vi "CheckData.vi"() -> ()   [LabVIEW 2019]
uses:
  Communication/TypeDef/#TypeDef_PropertiesToSave.ctl
  App/Global_Freq.vi
  <vilib>/Analysis/NI_AALBase.lvlib
  <vilib>/Analysis/baseanly.llb/Mean (DBL).vi
  <vilib>/Analysis/NI_AALPro.lvlib
  <vilib>/Analysis/5stat.llb/RMS (DBL).vi
  <vilib>/gmath/NI_Gmath.lvlib
panel:
  in  "Calc":bool
  in  "Tab Control":enum32{"Page 1", "Page 2", "Page 3"}(tab)
  out "Mean":dbl[][](graph)
  out "Corelation R^2":dbl[][](graph)
  out "RMS":dbl[][](graph)
  out "Corelation R":dbl[][](graph)
  out "Step":dbl format="%#_13g"
  out "TEST":cluster{"f0":dbl, "df":dbl, "magnitude":dbl[]}[](graph) caption="Power Spectrum TEST"
  out "POMIAR":cluster{"f0":dbl, "df":dbl, "magnitude":dbl[]}[](graph) caption="Power Spectrum POMIAR"
  out "Z":dbl[][](graph)
  out "Y":dbl[][](graph)
  out "X":dbl[][](graph)
  in  "Test Offset":i32
  in  "Pomiar Offset":i32
  in  "file path":path
  out "Poperties":T1
  in  "stop":bool
  in  "Lista_Archive":i32(listbox) caption="Lista pomiarów"
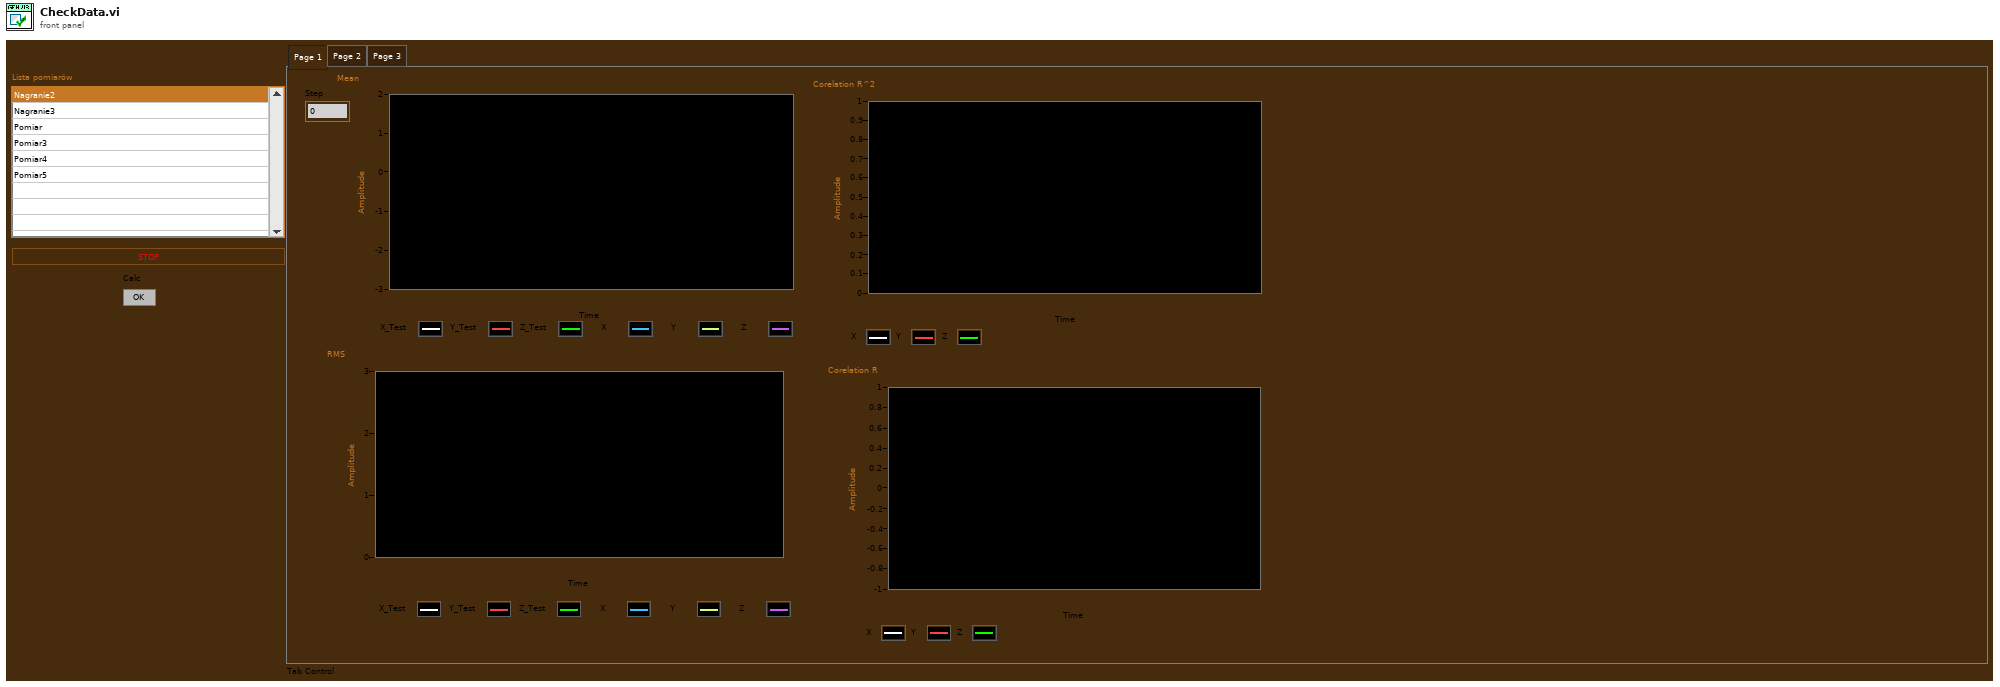
[diagram p1: front panel]
types:
  T1 = typedef "#TypeDef_PropertiesToSave.ctl" = cluster{"RMS values":dbl[], "Max":dbl[], "Min":dbl[], "A(8)":dbl[], "t":dbl, "A(8) Axis":dbl, "Aw":dbl[], "Ak 30min":dbl, "Ak_axis":i32, "Spec":cluster{"f0":dbl, "df":dbl, "magnitude":dbl[]}[]}
  T2 = enum16{"open", "open or create", "create or replace", "create", "open (read-only)"}
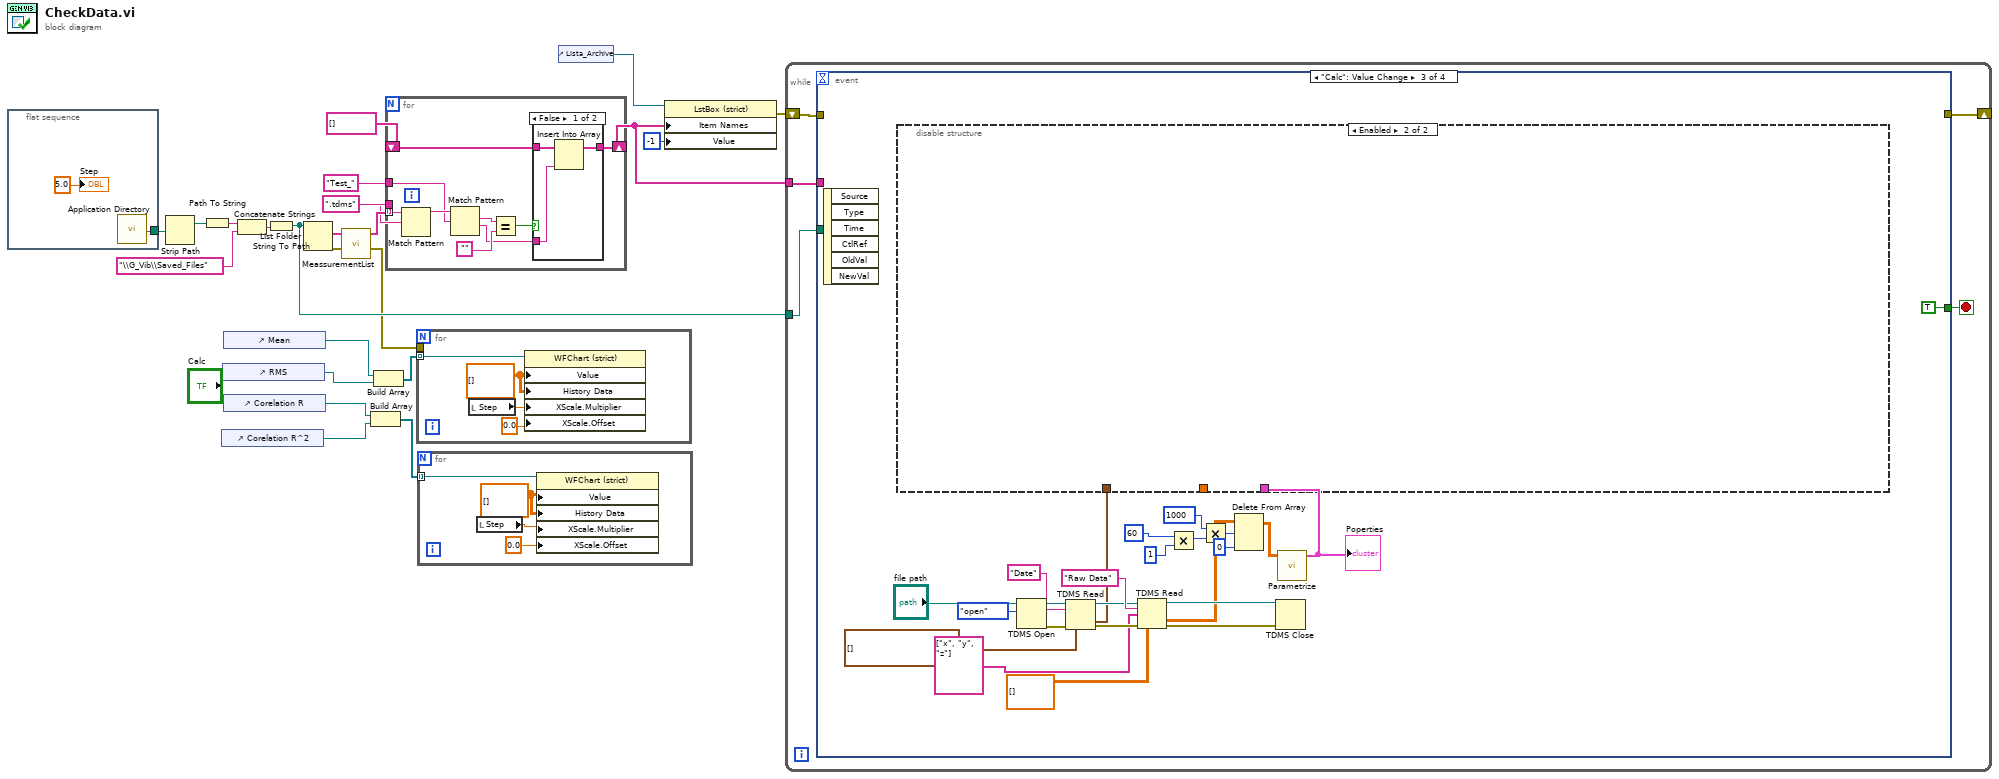
[diagram p0: block diagram]
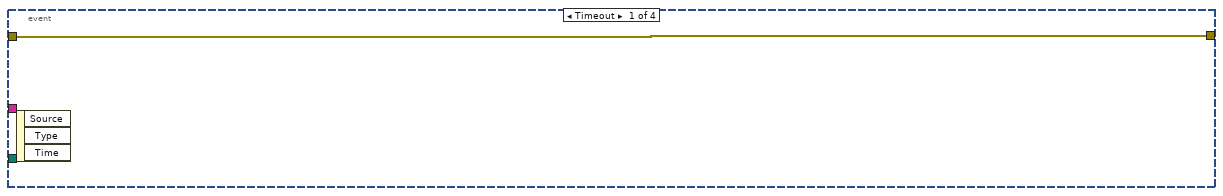
[diagram p2: hidden frame]
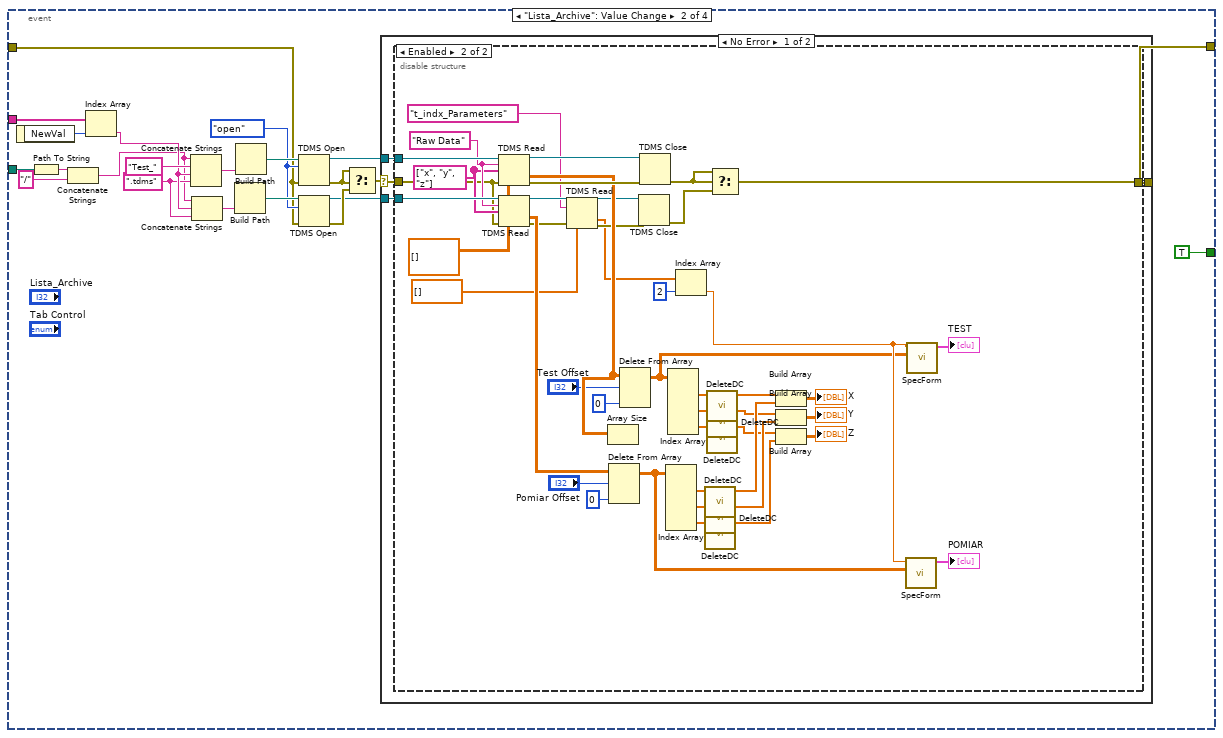
[diagram p3: hidden frame]
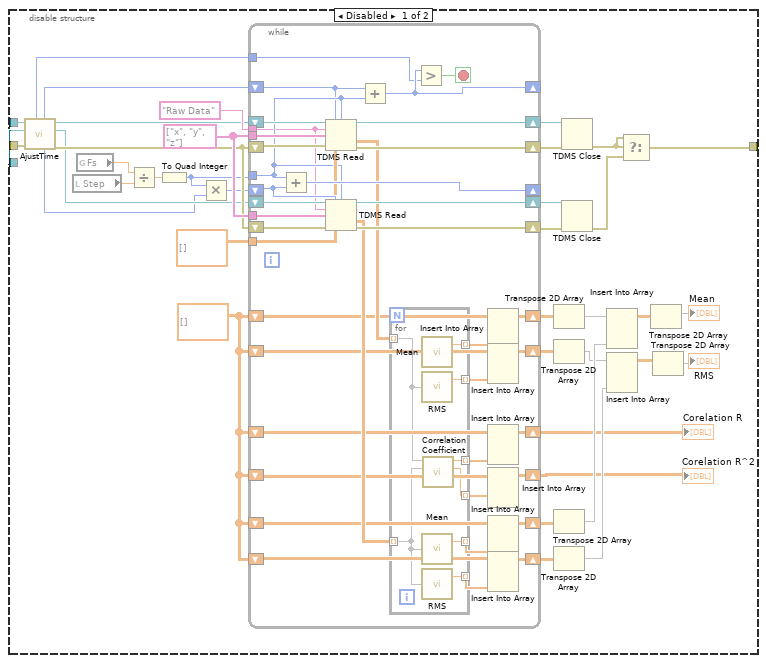
[diagram p4: hidden frame]
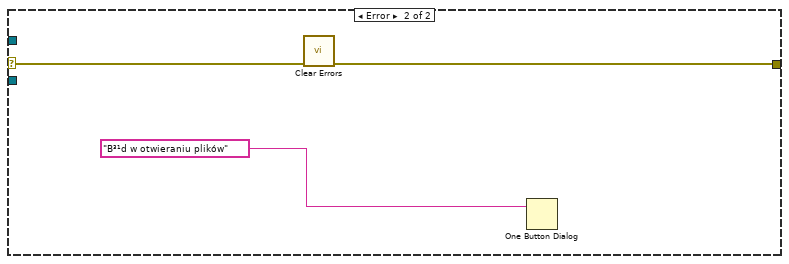
[diagram p5: hidden frame]
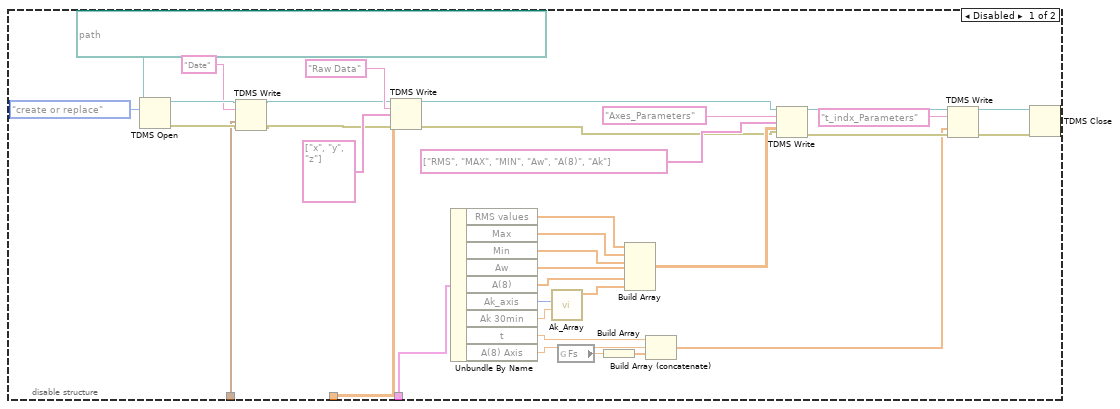
[diagram p6: hidden frame]
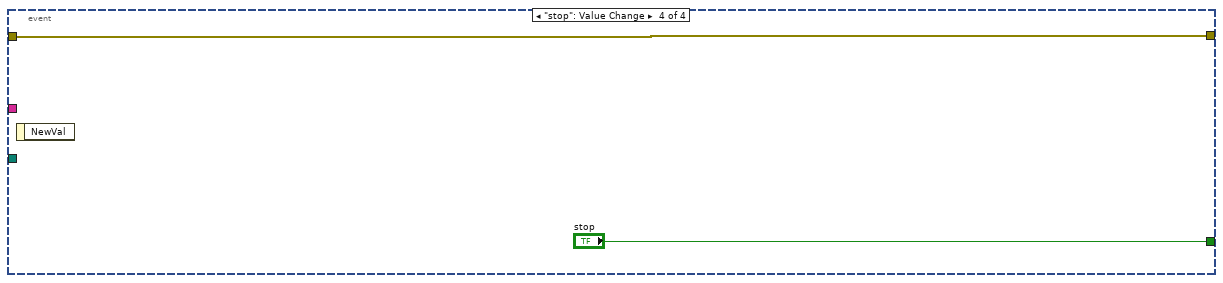
[diagram p7: hidden frame]
diagram:
  n1 = flat-sequence {
    tunnel: [w24] -> w2
    frame #0 {
      n2 = call <vilib>:"Application Directory.vi"() -> ("Application Directory"=w24:path)
      "Step" <- 5.0 ("Step")
    }
  }
  n3 = Strip Path(path=w2) -> (stripped path=w22:path)  [unwired: 1 out]
  n4 = Path To String(path=w22) -> (string=w21:string)
  n5 = control-ref of="Corelation R^2"() -> (w6:refnum<vi>)
  n6 = control-ref of="RMS"() -> (w8:refnum<vi>)
  n7 = control-ref of="Mean"() -> (w9:refnum<vi>)
  n8 = control-ref of="Corelation R"() -> (w7:refnum<vi>)
  n9 = Concatenate Strings(w21, "\\G_Vib\\Saved_Files" ("string")) -> (w20:string)
  n10 = String To Path(string=w20) -> (path=w10:path)
  n11 = List Folder(path=w10) -> (filenames=w18:string[], error out=w3:errorcluster)  [unwired: 3 in, 2 out]
  n12 = call "MeassurementList.vi"("filenames"=w18) -> ("ListaPomiarów"=w17:string[])  [unwired: 10 in]
  n13 = Build Array(w7, w6) -> (w4:refnum<vi>[])
  n14 = Build Array(w9, w8) -> (w5:refnum<vi>[])
  n15 = for {
    tunnel: w17 -> [w34] mode=indexing
    tunnel: ".tdms" -> [w33]
    tunnel: "Test_" ("regular expression") -> [w31]
    shift-right: [w26] -> w11
    shift-left: string[] [] -> [w25]
    n16 = Match Pattern(string=w34, regular expression=w33) -> (before substring=w32:string)  [unwired: 1 in, 3 out]
    n17 = Match Pattern(string=w32, regular expression=w31) -> (match substring=w30:string, after substring=w27:string)  [unwired: 1 in, 2 out]
    n18 = Equal?(x=w30, y="") -> (x = y?=w28:bool)
    n19 = case shown="False" w28 {
      tunnel: w27 -> [w37 _]
      tunnel: [w36 w38] -> w26
      tunnel: w25 -> [w35 w38]
      frame False {
        n20 = Insert Into Array(array=w35, new element=w37) -> (w36:string[])  [unwired: 1 in]
      }
      frame True {
      }
    }
  }
  n21 = for {
    tunnel: w5 -> [w42] mode=indexing
    tunnel: w3 -> [_]
    w40 = dbl[][] [] ("Value")
    n22 = local read "Step"() -> (w39:dbl)
    n23 = property class="WFChart (strict)"(reference=w42, "Value"=w40, "History Data"=w40, "XScale.Multiplier"=w39, "XScale.Offset"=0.0 ("X Scale.Offset and Multiplier:Offset")) -> ()  [unwired: 1 in, 2 out]
  }
  n24 = for {
    tunnel: w4 -> [w46] mode=indexing
    w44 = dbl[][] [] ("Value")
    n25 = local read "Step"() -> (w43:dbl)
    n26 = property class="WFChart (strict)"(reference=w46, "Value"=w44, "History Data"=w44, "XScale.Multiplier"=w43, "XScale.Offset"=0.0 ("X Scale.Offset and Multiplier:Offset")) -> ()  [unwired: 1 in, 2 out]
  }
  n27 = control-ref of="Lista_Archive"() -> (w13:refnum<vi>)
  n28 = property class="LstBox (strict)"(reference=w13, "Item Names"=w11, "Value"=-1) -> (error out=w12:errorcluster)  [unwired: 1 in, 1 out]
  n29 = while {
    tunnel: w11 -> [w50]
    tunnel: w10 -> [w49]
    shift-right: [w47] -> _
    shift-left: w12 -> [w48]
    stop <- w51 stop-if-true
    n30 = event shown="[2] \"Calc\": Value Change" {
      selector: _ -> [_ _ _ _]
      dyn-events: _ -> [_ _ _ _]
      timeout: _ -> [_ _ _ _]
      tunnel: [_ TRUE ("stop") TRUE ("stop") "stop"] -> w51
      tunnel: w50 -> [_ w74 _ _]
      tunnel: w49 -> [_ w72 _ _]
      tunnel: w48 -> [w52 w55 _ w272]
      tunnel: [w52 w54 _ w272] -> w47
      event Timeout {
        n31 = event-data() -> ()  [unwired: 1 in, 3 out]
      }
      event "Lista_Archive": Value Change {
        w61 = T2."open" ("operation (0:open)")
        w68 = ".tdms" ("string")
        n32 = event-data() -> ("NewVal"=w66:i32)  [unwired: 1 in]
        n33 = Path To String(path=w72) -> (string=w71:string)
        n34 = Concatenate Strings(w71, "/" ("string")) -> (w67:string)
        n35 = Index Array(array=w74, index=w66) -> (element=w69:string)
        n36 = Concatenate Strings(w67, "Test_" ("string"), w69, w68) -> (w65:string)
        n37 = Concatenate Strings(w67, w69, w68) -> (w64:string)
        n38 = Build Path(name or relative path=w64) -> (appended path=w62:path)  [unwired: 1 in]
        n39 = Build Path(name or relative path=w65) -> (appended path=w63:path)  [unwired: 1 in]
        n40 = TDMS Open(8:w55, 10:w61, 11:w63) -> (0:w60:errorcluster, 3:w57:refnum<k34>)  [unwired: 4 in]
        n41 = TDMS Open(8:w55, 10:w61, 11:w62) -> (0:w59:errorcluster, 3:w56:refnum<k34>)  [unwired: 4 in]
        n42 = Select(t=w60, s=w60, f=w59) -> (s? t:f=w58:errorcluster)
        n43 = case shown="No Error" w58 {
          selector: w58 -> [w77 w212]
          tunnel: w57 -> [w76 _]
          tunnel: w56 -> [w75 _]
          tunnel: [w78 w211] -> w54
          frame No Error {
            n44 = disable-structure shown="Enabled" {
              disable-tunnel: [w108 w183] -> w78
              disable-tunnel: w77 -> [w107 w205]
              disable-tunnel: w76 -> [w106 w209]
              disable-tunnel: w75 -> [w105 w208]
              frame Disabled {
                w101 = dbl[][] []
                w111 = string[] ["x", "y", "z"] ("channel name(s) in (Untitled)")
                n45 = call "AjustTime.vi"("error in (no error)"=w107, "Pomiar in"=w105, "Test in"=w106) -> ("error out"=w103:errorcluster, "Pomiar Out"=w102:refnum<k34>, "Test Out"=w104:refnum<k34>, "First Pomiar"=w81:i64, "FirstTest"=w80:i64, "End"=w82:i64)  [unwired: 3 in]
                n46 = local read "Step"() -> (w83:dbl)
                n47 = global read "Global_Freq.vi" "Fs"() -> (w85:dbl)
                n48 = Divide(x=w85, y=w83) -> (x/y=w84:dbl)
                n49 = To Quad Integer(1:w84) -> (0:w90:i64)
                n50 = Multiply(x=w90, y=w81) -> (x*y=w86:i64)
                n51 = while {
                  shift-right: [w153] -> _
                  shift-left: w86 -> [w152]
                  shift-right: [w150] -> w114
                  shift-left: w103 -> [w154]
                  shift-right: [w151] -> w116
                  shift-left: w103 -> [w155]
                  tunnel: dbl[][] [] ("element") -> [w148]
                  tunnel: "Raw Data" ("group name in (Untitled)") -> [w123]
                  tunnel: w111 -> [w147]
                  tunnel: w111 -> [w146]
                  shift-right: [w138] -> w87
                  shift-left: w101 -> [w137]
                  shift-right: [w136] -> w100
                  shift-left: w101 -> [w135]
                  shift-right: [w134] -> w89
                  shift-left: w101 -> [w133]
                  shift-right: [w132] -> w88
                  shift-left: w101 -> [w131]
                  shift-right: [w130] -> w99
                  shift-left: w101 -> [w129]
                  shift-right: [w128] -> w98
                  shift-left: w101 -> [w127]
                  tunnel: w90 -> [w125]
                  shift-right: [w120] -> _
                  shift-left: w80 -> [w121]
                  shift-right: [w149] -> w115
                  shift-left: w102 -> [w126]
                  shift-right: [w124] -> w117
                  shift-left: w104 -> [w156]
                  tunnel: w82 -> [w119]
                  stop <- w118 stop-if-true
                  n52 = Add(x=w125, y=w152) -> (x+y=w153:i64)
                  n53 = TDMS Read(0:w156, 1:w121, 2:w125, 5:w123, 7:w147, 11:w155, 12:w148) -> (4:w124:refnum<k34>, 10:w140:dbl[][], 15:w151:errorcluster)  [unwired: 1 in, 3 out]
                  n54 = TDMS Read(0:w126, 1:w152, 2:w125, 5:w123, 7:w146, 11:w154, 12:w148) -> (4:w149:refnum<k34>, 10:w139:dbl[][], 15:w150:errorcluster)  [unwired: 1 in, 3 out]
                  n55 = Add(x=w121, y=w125) -> (x+y=w120:i64)
                  n56 = for {
                    tunnel: w140 -> [w164] mode=indexing
                    tunnel: w139 -> [w163] mode=indexing
                    tunnel: [w157] -> w122 mode=indexing
                    tunnel: [w162] -> w145 mode=indexing
                    tunnel: [w161] -> w144 mode=indexing
                    tunnel: [w160] -> w143 mode=indexing
                    tunnel: [w159] -> w142 mode=indexing
                    tunnel: [w158] -> w141 mode=indexing
                    n57 = call-poly <vilib>:"Mean.vi"("X"=w164) -> ("mean"=w157:dbl)  [unwired: 1 out]
                    n58 = call-poly <vilib>:"RMS.vi"("X"=w164) -> ("rms value"=w162:dbl)  [unwired: 1 out]
                    n59 = call-poly <vilib>:"Mean.vi"("X"=w163) -> ("mean"=w161:dbl)  [unwired: 1 out]
                    n60 = call-poly <vilib>:"RMS.vi"("X"=w163) -> ("rms value"=w160:dbl)  [unwired: 1 out]
                    n61 = call <vilib>:"Correlation Coefficient.vi"("Y"=w163, "X"=w164) -> ("r^2"=w158:dbl, "correlation coefficient r"=w159:dbl)  [unwired: 8 in]
                  }
                  n62 = Greater?(x=w120, y=w119) -> (0:w118:bool)
                  n63 = Insert Into Array(array=w137, new element=w122) -> (w138:dbl[][])  [unwired: 2 in]
                  n64 = Insert Into Array(array=w135, new element=w145) -> (w136:dbl[][])  [unwired: 2 in]
                  n65 = Insert Into Array(array=w133, new element=w142) -> (w134:dbl[][])  [unwired: 2 in]
                  n66 = Insert Into Array(array=w131, new element=w141) -> (w132:dbl[][])  [unwired: 2 in]
                  n67 = Insert Into Array(array=w129, new element=w144) -> (w130:dbl[][])  [unwired: 2 in]
                  n68 = Insert Into Array(array=w127, new element=w143) -> (w128:dbl[][])  [unwired: 2 in]
                }
                "Corelation R" <- w89
                "Corelation R^2" <- w88
                n69 = Transpose 2D Array(2D array=w87) -> (transposed array=w96:dbl[][])
                n70 = Transpose 2D Array(2D array=w100) -> (transposed array=w95:dbl[][])
                n71 = Transpose 2D Array(2D array=w99) -> (transposed array=w97:dbl[][])
                n72 = Transpose 2D Array(2D array=w98) -> (transposed array=w94:dbl[][])
                n73 = TDMS Close(8:w116, 11:w117) -> (0:w110:errorcluster)  [unwired: 1 out]
                n74 = TDMS Close(8:w114, 11:w115) -> (0:w109:errorcluster)  [unwired: 1 out]
                n75 = Insert Into Array(array=w96, new element=w97) -> (w79:dbl[][])  [unwired: 2 in]
                n76 = Insert Into Array(array=w95, new element=w94) -> (w92:dbl[][])  [unwired: 2 in]
                n77 = Select(t=w110, s=w110, f=w109) -> (s? t:f=w108:errorcluster)
                n78 = Transpose 2D Array(2D array=w79) -> (transposed array=→"Mean":dbl[][])
                n79 = Transpose 2D Array(2D array=w92) -> (transposed array=→"RMS":dbl[][])
              }
              frame Enabled {
                w204 = dbl[][] [] ("element")
                w206 = string[] ["x", "y", "z"] ("channel name(s) in (Untitled)")
                w207 = "Raw Data" ("group name in (Untitled)")
                n80 = TDMS Read(0:w209, 5:w207, 7:w206, 11:w205, 12:w204) -> (4:w185:refnum<k34>, 10:w182:dbl[][], 15:w184:errorcluster)  [unwired: 3 in, 3 out]
                n81 = TDMS Read(0:w208, 5:w207, 7:w206, 11:w205, 12:w204) -> (4:w177:refnum<k34>, 10:w188:dbl[][], 15:w175:errorcluster)  [unwired: 3 in, 3 out]
                n82 = TDMS Read(0:w177, 5:"t_indx_Parameters" ("group name in (Untitled)"), 11:w175, 12:dbl[] [] ("element")) -> (4:w176:refnum<k34>, 10:w171:dbl[], 15:w174:errorcluster)  [unwired: 4 in, 3 out]
                n83 = Array Size(array=w182) -> ()  [unwired: 1 out]
                n84 = Delete From Array(array=w188, length="Pomiar Offset", index (col)=0 ("index (row)")) -> (array with subset deleted=w169:dbl[][])  [unwired: 1 in, 1 out]
                n85 = Delete From Array(array=w182, length="Test Offset", index (col)=0 ("index (row)")) -> (array with subset deleted=w166:dbl[][])  [unwired: 1 in, 1 out]
                n86 = TDMS Close(8:w174, 11:w176) -> (0:w186:errorcluster)  [unwired: 1 out]
                n87 = TDMS Close(8:w184, 11:w185) -> (0:w187:errorcluster)  [unwired: 1 out]
                n88 = Index Array(array=w169) -> (element #1=w200:dbl[], element #2=w199:dbl[], element #3=w198:dbl[])  [unwired: 6 in]
                n89 = Index Array(array=w166) -> (element #1=w203:dbl[], element #2=w202:dbl[], element #3=w201:dbl[])  [unwired: 6 in]
                n90 = Index Array(array=w171, index=2) -> (element=w167:dbl)
                n91 = call "DeleteDC.vi"("element"=w200) -> ("Array"=w196:dbl[])  [unwired: 10 in]
                n92 = call "DeleteDC.vi"("element"=w199) -> ("Array"=w193:dbl[])  [unwired: 10 in]
                n93 = call "DeleteDC.vi"("element"=w198) -> ("Array"=w190:dbl[])  [unwired: 10 in]
                n94 = call "DeleteDC.vi"("element"=w203) -> ("Array"=w197:dbl[])  [unwired: 10 in]
                n95 = call "DeleteDC.vi"("element"=w202) -> ("Array"=w194:dbl[])  [unwired: 10 in]
                n96 = call "DeleteDC.vi"("element"=w201) -> ("Array"=w191:dbl[])  [unwired: 10 in]
                n97 = Select(t=w187, s=w187, f=w186) -> (s? t:f=w183:errorcluster)
                n98 = Build Array(w197, w196) -> (→"X":dbl[][])
                n99 = Build Array(w194, w193) -> (→"Y":dbl[][])
                n100 = Build Array(w191, w190) -> (→"Z":dbl[][])
                n101 = call "SpecForm.vi"("Data"=w169, "Fs"=w167) -> ("Power Spectrum / PSD"=→"POMIAR":cluster{"f0":dbl, "df":dbl, "magnitude":dbl[]}[])  [unwired: 9 in]
                n102 = call "SpecForm.vi"("Data"=w166, "Fs"=w167) -> ("Power Spectrum / PSD"=→"TEST":cluster{"f0":dbl, "df":dbl, "magnitude":dbl[]}[])  [unwired: 9 in]
              }
            }
          }
          frame Error {
            n103 = call <vilib>:"Clear Errors.vi"("error in (no error)"=w212) -> ("error out"=w211:errorcluster)  [unwired: 5 in, 1 out]
            n104 = One Button Dialog(message="B³¹d w otwieraniu plików") -> ()  [unwired: 1 in, 1 out]
          }
        }
      }
      event "Calc": Value Change {
        n105 = event-data() -> ()  [unwired: 1 in, 6 out]
        n106 = TDMS Open(10:T2."open" ("operation (0:open)"), 11:"file path") -> (0:w229:errorcluster, 3:w230:refnum<k34>)  [unwired: 5 in]
        n107 = TDMS Read(0:w230, 5:"Date" ("group name in"), 11:w229, 12:timestamp[] [] ("appended array")) -> (4:w228:refnum<k34>, 10:w223:timestamp[], 15:w227:errorcluster)  [unwired: 4 in, 3 out]
        n108 = TDMS Read(0:w228, 5:"Raw Data" ("group name in"), 7:string[] ["x", "y", "z"] ("channel name(s) in"), 11:w227, 12:dbl[][] [] ("Raw Data")) -> (4:w231:refnum<k34>, 10:w214:dbl[][], 15:w236:errorcluster)  [unwired: 3 in, 3 out]
        n109 = Multiply(x=60, y=1) -> (x*y=w216:i32)
        n110 = Multiply(x=1000 ("length"), y=w216) -> (x*y=w219:i32)
        n111 = Delete From Array(array=w214, length=w219, index (col)=0 ("disabled index (col)")) -> (array with subset deleted=w213:dbl[][])  [unwired: 1 in, 1 out]
        n112 = TDMS Close(8:w236, 11:w231) -> ()  [unwired: 2 out]
        n113 = call "Parametrize.vi"("Raw Data"=w213) -> ("Poperties"=w233:T1)  [unwired: 10 in]
        "Poperties" <- w233
        n114 = disable-structure shown="Enabled" {
          disable-tunnel: w233 -> [w252 _]
          disable-tunnel: _ -> [w247 _]
          disable-tunnel: w223 -> [w239 _]
          frame Disabled {
            n115 = TDMS Open(10:T2."create or replace" ("operation (0:open)"), 11:path "D:/Materiały/#Studia/IA/#_MAGISTERSKIE/Magisterka/G_Vib/Saved_Files/Pom2.tdms" ("base path")) -> (0:w240:errorcluster, 3:w238:refnum<k34>)  [unwired: 5 in]
            n116 = TDMS Write(0:w238, 5:"Date" ("group name in"), 9:w239, 11:w240) -> (4:w242:refnum<k34>, 15:w241:errorcluster)  [unwired: 2 in, 2 out]
            n117 = TDMS Write(0:w242, 5:"Raw Data" ("group name in"), 7:string[] ["x", "y", "z"] ("channel name(s) in"), 9:w247, 11:w241) -> (4:w248:refnum<k34>, 15:w249:errorcluster)  [unwired: 1 in, 2 out]
            n118 = Unbundle By Name(w252) -> ("RMS values"=w259:dbl[], "Max"=w260:dbl[], "Min"=w261:dbl[], "Aw"=w267:dbl[], "A(8)"=w266:dbl[], "Ak_axis"=w256:i32, "Ak 30min"=w255:dbl, "t"=w264:dbl, "A(8) Axis"=w263:dbl)
            n119 = call "Ak_Array.vi"("Ak 30min"=w255, "Ak_axis"=w256) -> ("Ak Aray"=w257:dbl[])  [unwired: 9 in]
            n120 = global read "Global_Freq.vi" "Fs"() -> (w254:dbl)
            n121 = Build Array(w254) -> (w253:dbl[])
            n122 = Build Array(w259, w260, w261, w267, w266, w257) -> (w265:dbl[][])
            n123 = Build Array (concatenate)(w264, w263, w253) -> (w262:dbl[])
            n124 = TDMS Write(0:w248, 5:"Axes_Parameters" ("group name in (Untitled)"), 7:string[] ["RMS", "MAX", "MIN", "Aw", "A(8)", "Ak"] ("channel name(s) in (Untitled)"), 9:w265, 11:w249) -> (4:w271:refnum<k34>, 15:w270:errorcluster)  [unwired: 1 in, 2 out]
            n125 = TDMS Write(0:w271, 5:"t_indx_Parameters" ("group name in (Untitled)"), 9:w262, 11:w270) -> (4:w251:refnum<k34>, 15:w250:errorcluster)  [unwired: 2 in, 2 out]
            n126 = TDMS Close(8:w250, 11:w251) -> ()  [unwired: 2 out]
          }
          frame Enabled {
          }
        }
      }
      event "stop": Value Change {
        n127 = event-data() -> ()  [unwired: 1 in, 1 out]
      }
    }
  }
